vi "Data-to-string.vi"(1 "string":string="Comments: Bla-Bla", 2 "wavelength":dbl[](array[numeric]), 3 "timedelay":dbl[](array[numeric]), 4 "DATA":dbl[][](array[numeric])) -> (0 "resulted string":string)   [LabVIEW 2015]
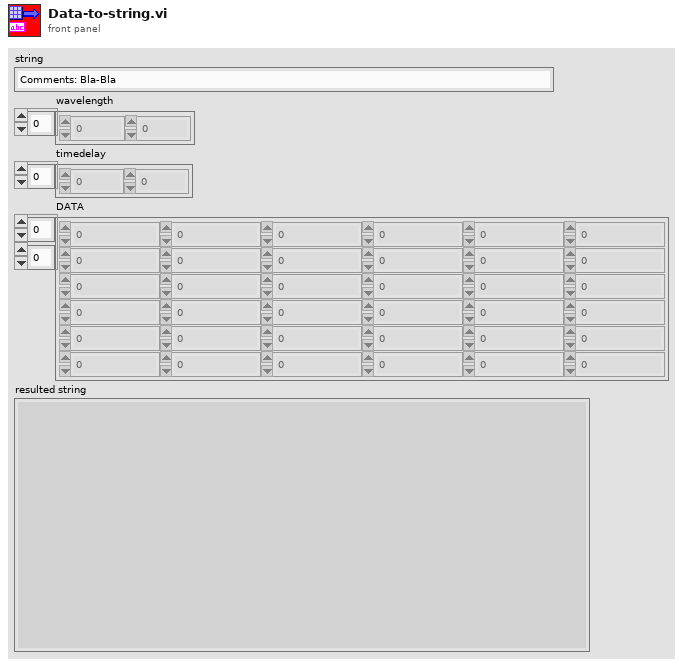
[diagram p1: front panel]
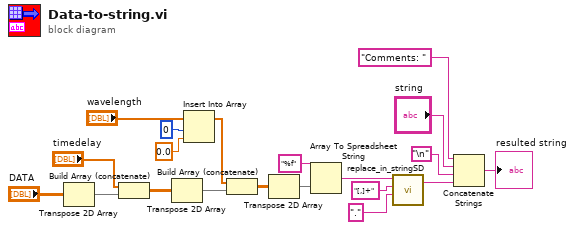
[diagram p0: block diagram]
diagram:
  n1 = Transpose 2D Array(2D array="DATA") -> (transposed array=w4:dbl[][])
  n2 = Build Array (concatenate)("timedelay", w4) -> (w6:dbl[][])
  n3 = Transpose 2D Array(2D array=w6) -> (transposed array=w15:dbl[][])
  n4 = Insert Into Array(array="wavelength", index=0, new element=0.0 ("new element/subarray")) -> (w16:dbl[])
  n5 = Build Array (concatenate)(w16, w15) -> (w3:dbl[][])
  n6 = Transpose 2D Array(2D array=w3) -> (transposed array=w2:dbl[][])
  n7 = Array To Spreadsheet String(array=w2, 3:"%f" ("format string")) -> (spreadsheet string=w10:string)  [unwired: 1 in]
  n8 = call "replace_in_stringSD.vi"("replaced to.."=".", "characters to replace"="[,]+", "input string"=w10) -> ("output string"=w7:string)  [unwired: 1 in, 1 out]
  n9 = Concatenate Strings("Comments: " ("string"), "string", "\n", w7) -> (→"resulted string":string)
